vi "DBL-round to 2 decimal places.vi"(8 "error in (no error)":errorcluster, 11 "Number in":dbl format="%.10g") -> (0 "error out":errorcluster, 2 "Number out (rounded to two decimals)":string, 3 "Number out (rounded to two decimals)":dbl format="%.2f")   [LabVIEW 2021, in "Numeric Utilities.lvlib"]
uses:
  Numeric Utilities.lvlib
panel:
  # "Development\ncontrols/indicators useful for development and testing, but which are not outputs of the VI"
  # "Input\nInputs to the VI"
  # "Output\nOutputs of the VI"
  # "Description\n\nBlank VI with error handling case. \n\nSummarize the use of this VI in this space."
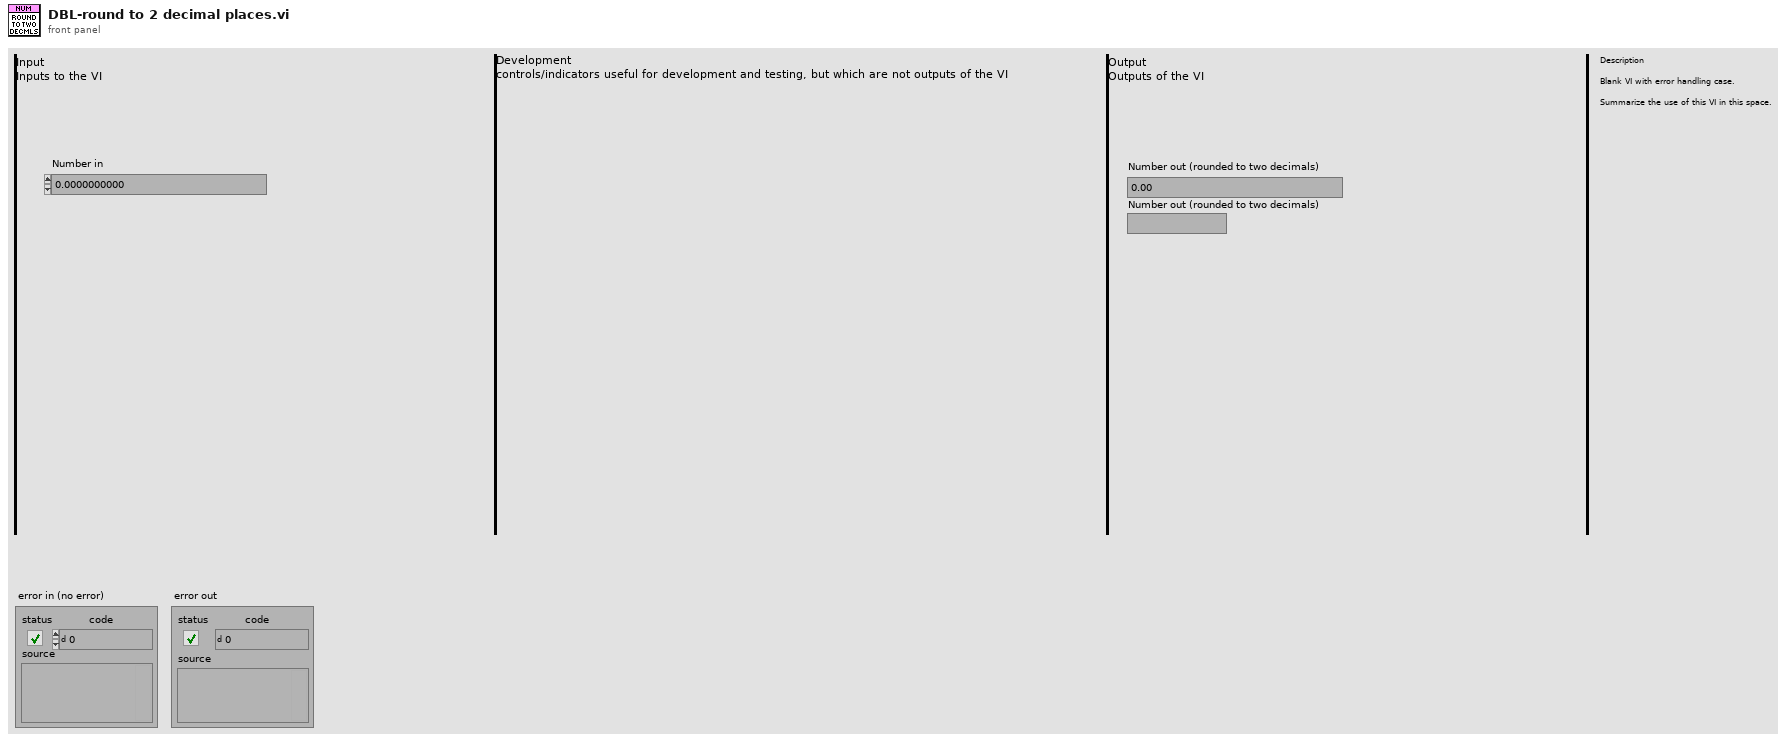
[diagram p1: front panel]
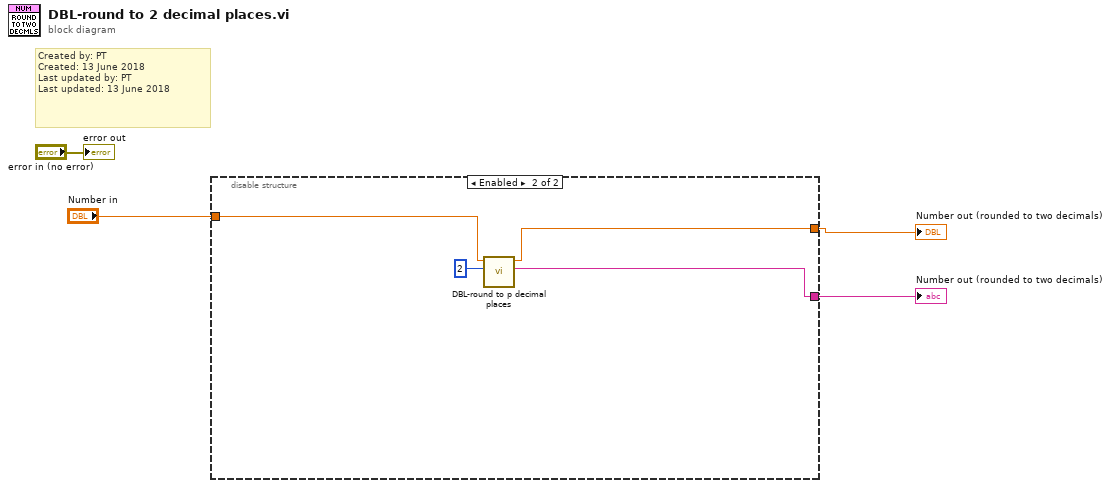
[diagram p0: block diagram]
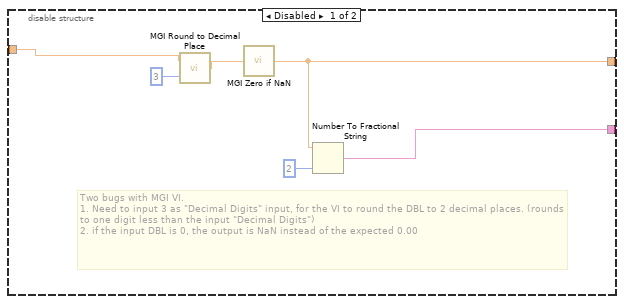
[diagram p2: hidden frame]
diagram:
  # "Created by: PT\nCreated: 13 June 2018\nLast updated by: PT\nLast updated: 13 June 2018"
  n1 = disable-structure shown="Enabled" {
    disable-tunnel: "Number in" -> [w7 w14]
    disable-tunnel: [w6 w12] -> w2
    disable-tunnel: [w5 w11] -> w1
    frame Disabled {
      # "Two bugs with MGI VI.\n1. Need to input 3 as \"Decimal Digits\" input, for the VI to round the DBL to 2 decimal places. (rounds to one digit less than the input \"Decimal Digits\")\n2. if the input DBL is 0, the output is NaN instead of the expected 0.00"
      n2 = call <userlib>:"MGI Round to Decimal Place.vi"("Decimal Digits"=3, "Number"=w7) -> ("Rounded"=w9:dbl)  [unwired: 1 in]
      n3 = call <userlib>:"MGI Zero if NaN.vi"("Number In"=w9) -> ("Number Out"=w6:dbl)
      n4 = Number To Fractional String(number=w6, precision (6)=i16 2) -> (F-format string=w5:string)  [unwired: 2 in]
    }
    frame Enabled {
      n5 = call "DBL-round to p decimal places.vi"("p = desired precision = number of digits after decimal point (dflt=2)"=u32 2 ("n = desired precision = number of digits after decimal point (dflt=2)"), "x = number in"=w14) -> ("Number out (rounded to p digits after decimal point)"=w11:string, "x= number out (rounded to p digits after decimal point)"=w12:dbl)  [unwired: 7 in, 1 out]
    }
  }
  "Number out (rounded to two decimals)" <- w2
  "Number out (rounded to two decimals)" <- w1
  "error out" <- "error in (no error)"
